vi "Reset.vi"(11 "file handler in":refnum<class "File Handler.lvclass">) -> (2 "successful?":bool, 3 "file handler out":refnum<class "File Handler.lvclass">)   [LabVIEW 2024, in "Logging.lvlib" / "File Handler.lvclass"]
uses:
  File Handler.lvclass
panel:
  # "Connector Pane"
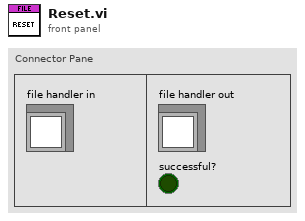
[diagram p1: front panel]
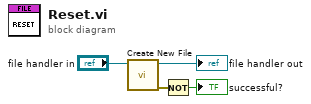
[diagram p0: block diagram]
diagram:
  n1 = call "Create New File.vi"("file handler in"="file handler in") -> ("error out"=w2:errorcluster, "file handler out"=→"file handler out":refnum<class "File Handler.lvclass">)  [unwired: 9 in]
  n2 = Not(x=w2) -> (.not. x?=→"successful?":bool)
